vi "Simulation.CalcNextIteration.vi"(0 "Simulation in":refnum<class "Simulation.lvclass">, 1 "SimMode":T1, 5 "error in (no error)":errorcluster) -> (14 "Simulation out":refnum<class "Simulation.lvclass">, 19 "error out":errorcluster)   [LabVIEW 2016, in "Simulation.lvclass"]
uses:
  Simulation.lvclass
  SimModes.ctl
  Simulation.lvclass/Simulation.ctl
  Modell/Sondenmodell/Sondenmodell.lvclass/Sondenmodell.ctl
  Modell/Hausmodell/Hausmodell.lvclass/Hausmodell.ctl
  Modell/Umgebung/Umgebung.lvclass/Umgebung.ctl
  Modell/Hausmodell/Hausmodell.lvclass
  Modell/Sondenmodell/Sondenmodell.lvclass
  Modell/Umgebung/Umgebung.lvclass
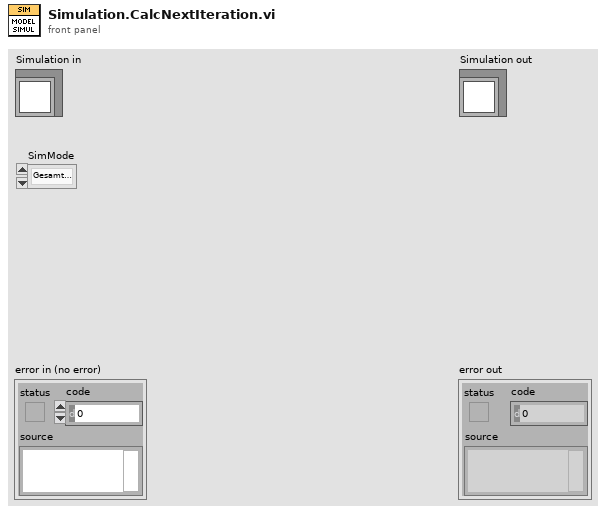
[diagram p1: front panel]
types:
  T1 = typedef "Simulation.lvclass/SimModes.ctl" = enum16{"Gesamtmodell", "HausOnly", "SondeOnly", "WPOnly"}
  T2 = typedef "Sondenmodell.lvclass/Sondenmodell.Zustandsgrössen.ctl" = cluster{"Erdtemperatur [°C]":dbl, "Rücklauftemperatur Solekreislauf [°C]":dbl}
  T3 = typedef "Hausmodell.lvclass/Hausmodell.Zustandsgrössen.ctl" = cluster{"Raumtemperatur [°C]":dbl, "Bodentemperatur [°C]":dbl, "Rücklauftemperatur Heizkreislauf [°C]":dbl}
  T4 = typedef "Umgebung.lvclass/Umgebung.Zustandsgrössen.ctl" = cluster{"Aussentemperatur [°C]":dbl, "Aussentemperatur [°C] Manuell":dbl, "Tag":dbl, "Stunde":dbl, "Minute":dbl, "Sekunden":dbl, "Strahlungsleistung [W/m2]":dbl, "Solare Gewinne [W/m2]":dbl, "Solare Gewinne [W/m2] Manuell":dbl, "Manuelle Eingabe On/Off":bool}
  T5 = typedef "Wärmepumpe.lvclass/Wärmepumpe.Zustandsgrössen.ctl" = cluster{"Vorlauftemperatur Heizkreislauf[°C]":dbl, "Vorlauftemperatur Solekreislauf[°C]":dbl, "Heizleistung [W]":dbl, "Kälteleistung [W]":dbl, "Verdichter 1":bool, "Verdichter 2":bool}
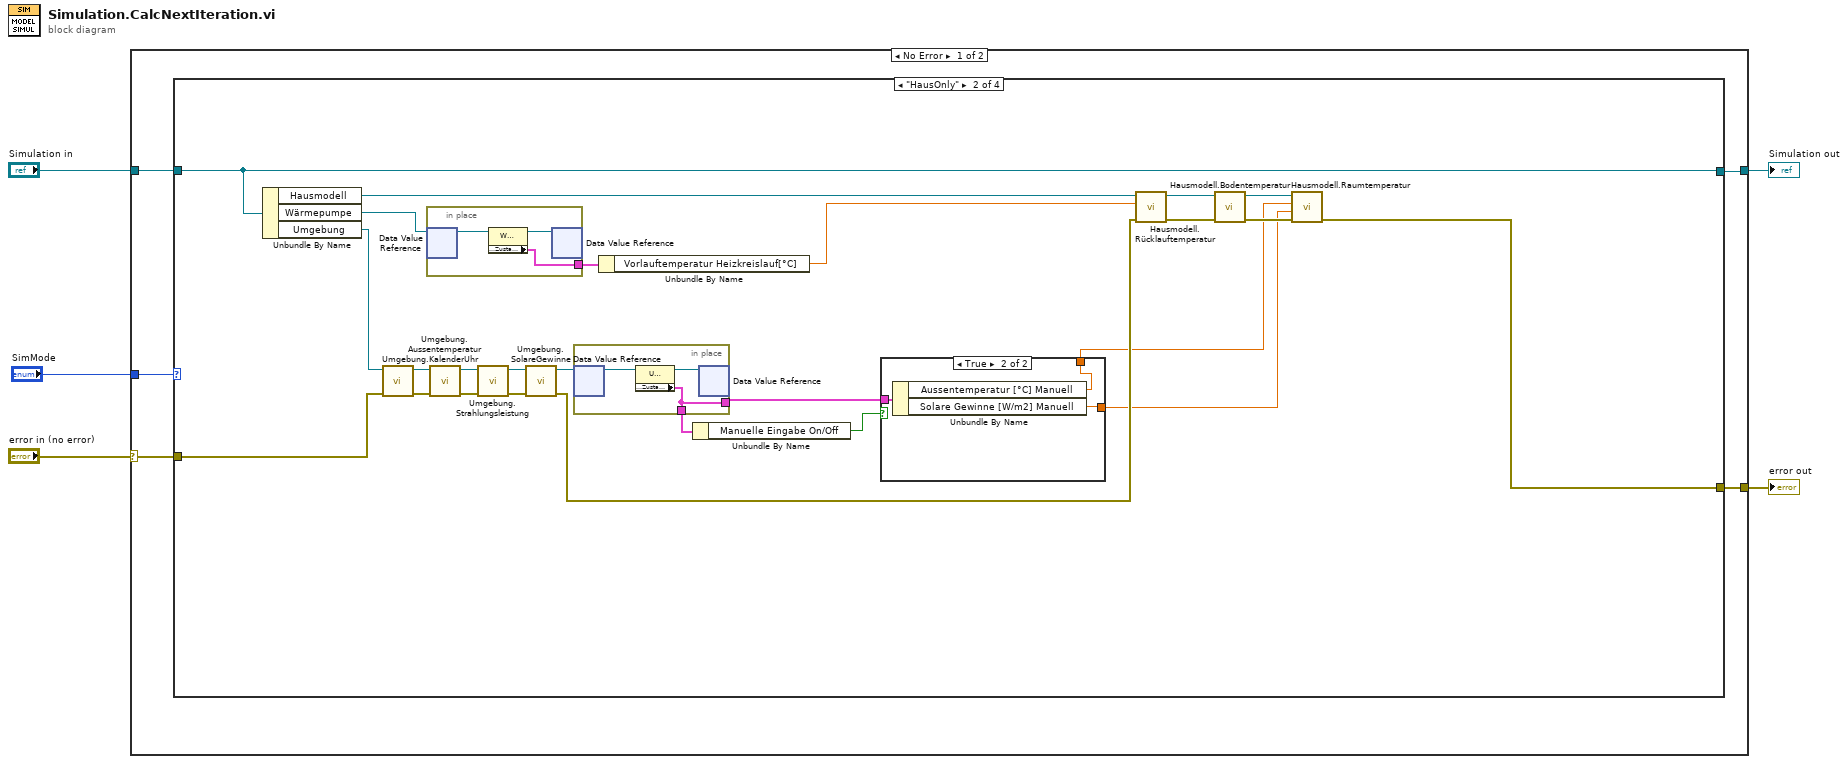
[diagram p0: block diagram]
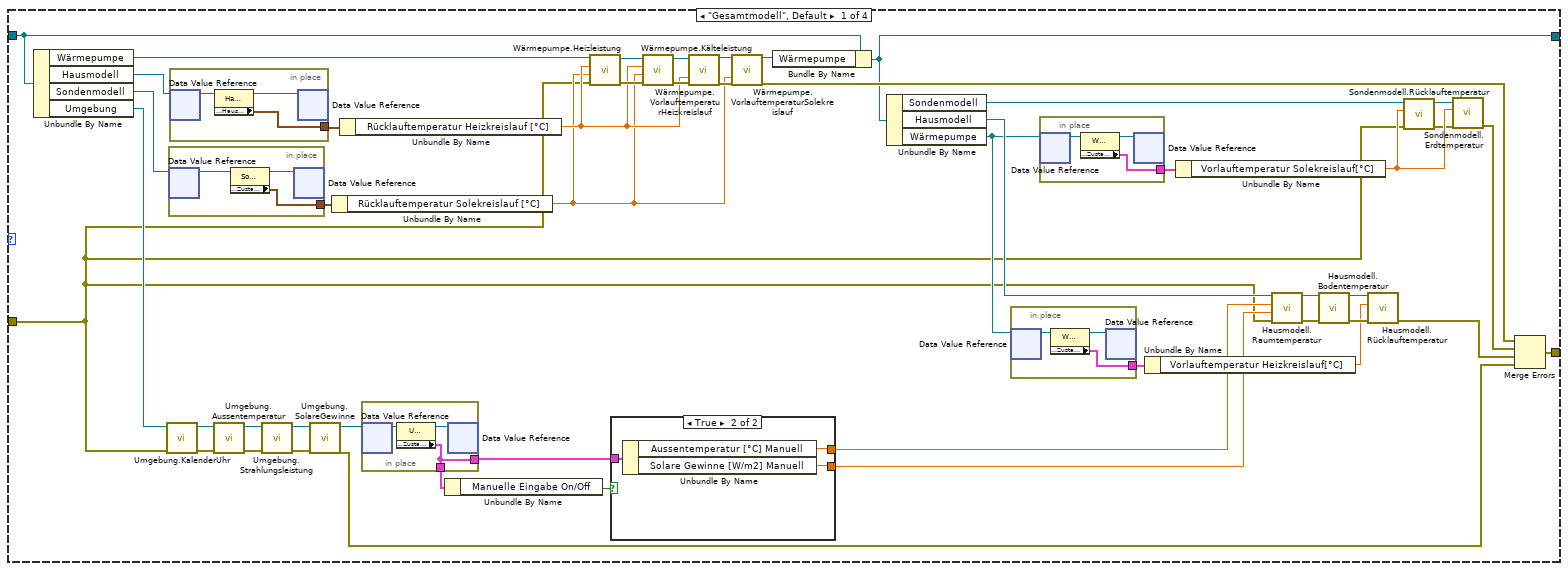
[diagram p2: hidden frame]
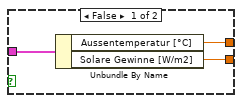
[diagram p3: hidden frame]
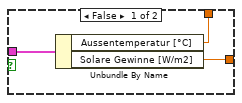
[diagram p4: hidden frame]
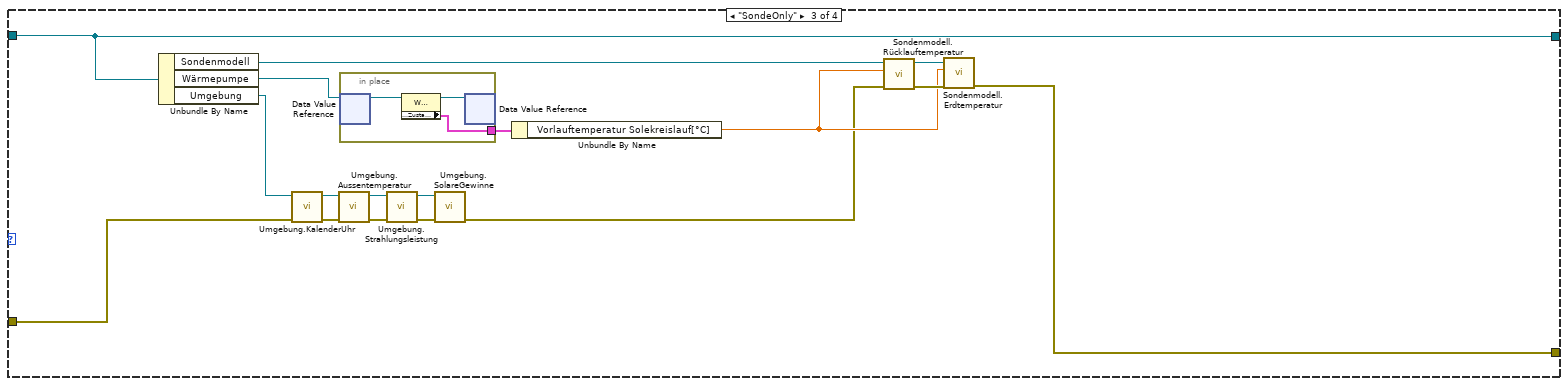
[diagram p5: hidden frame]
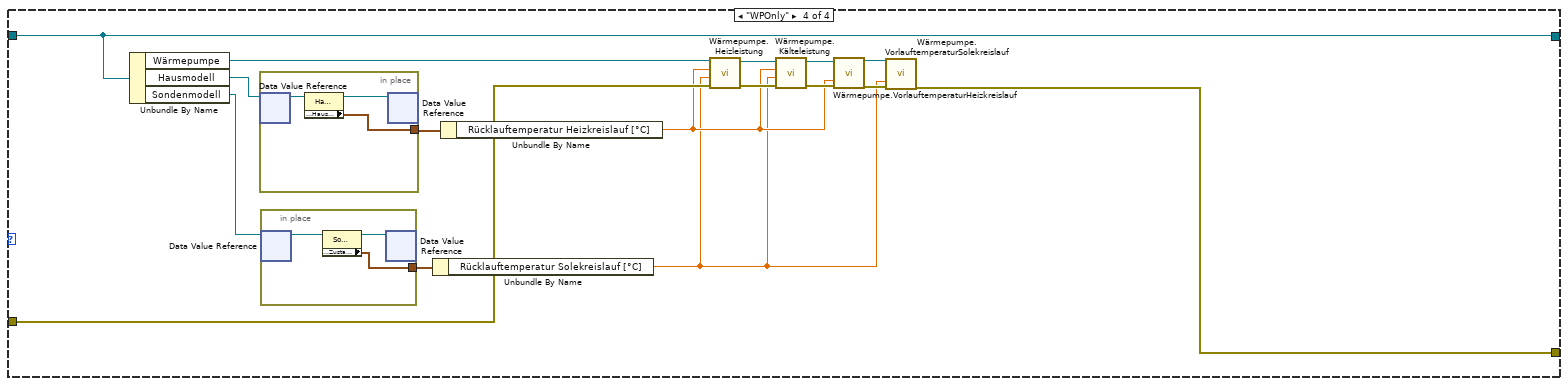
[diagram p6: hidden frame]
diagram:
  n1 = case shown="No Error" "error in (no error)" {
    selector: "error in (no error)" -> [w10 w160]
    tunnel: [w8 w160] -> w4
    tunnel: [w9 w159] -> w2
    tunnel: "Simulation in" -> [w7 w159]
    tunnel: "SimMode" -> [w6 _]
    frame No Error {
      n2 = case shown="\"HausOnly\"" w6 {
        tunnel: w10 -> [w13 w101 w118 w141]
        tunnel: [w23 w104 w131 w150] -> w9
        tunnel: [w34 w89 w127 w139] -> w8
        tunnel: w7 -> [w24 w104 w131 w150]
        frame "Gesamtmodell", Default {
          n3 = Unbundle By Name(w24) -> ("Wärmepumpe"=w50:refnum<data-value>, "Hausmodell"=w58:refnum<data-value>, "Sondenmodell"=w57:refnum<data-value>, "Umgebung"=w35:refnum<data-value>)
          n4 = call "Umgebung.KalenderUhr.vi"("Error in"=w13, "Umgebung in"=w35) -> ("Error out"=w42:errorcluster, "Umgebung out"=w45:refnum<data-value>)  [unwired: 8 in]
          n5 = in-place {
            in-place-border: [w74] -> w52
            n6 = in-place-dvr #1(w57) -> (w76:refnum<class "Sondenmodell.lvclass">)  [unwired: 1 out]
            n7 = property class="Sondenmodell.lvclass"(reference=w76) -> (reference out=w75:refnum<class "Sondenmodell.lvclass">, "Accessors:Sondenmodell.Zustandsgrössen"=w74:T2)  [unwired: 1 in, 1 out]
            n8 = in-place-dvr #1(w75) -> ()  [unwired: 2 out]
          }
          n9 = in-place {
            in-place-border: [w77] -> w51
            n10 = in-place-dvr #2(w58) -> (w79:refnum<class "Hausmodell.lvclass">)  [unwired: 1 out]
            n11 = property class="Hausmodell.lvclass"(reference=w79) -> (reference out=w78:refnum<class "Hausmodell.lvclass">, "Accessors:Zustandsgrössen.Hausmodell"=w77:T3)  [unwired: 1 in, 1 out]
            n12 = in-place-dvr #2(w78) -> ()  [unwired: 2 out]
          }
          n13 = call "Umgebung.Aussentemperatur.vi"("Error in"=w42, "Umgebung in"=w45) -> ("Error out"=w41:errorcluster, "Umgebung out"=w44:refnum<data-value>)  [unwired: 8 in]
          n14 = call "Umgebung.Strahlungsleistung.vi"("Error in"=w41, "Umgebung in"=w44) -> ("Error out"=w40:errorcluster, "Umgebung out"=w43:refnum<data-value>)  [unwired: 8 in]
          n15 = call "Umgebung.SolareGewinne.vi"("Error in"=w40, "Umgebung in"=w43) -> ("Error out"=w33:errorcluster, "Umgebung out"=w39:refnum<data-value>)  [unwired: 8 in]
          n16 = Unbundle By Name(w52) -> ("Rücklauftemperatur Solekreislauf [°C]"=w46:dbl)
          n17 = Unbundle By Name(w51) -> ("Rücklauftemperatur Heizkreislauf [°C]"=w47:dbl)
          n18 = in-place {
            in-place-border: [w71] -> w36
            in-place-border: [w71] -> w38
            n19 = in-place-dvr #3(w39) -> (w73:refnum<class "Umgebung.lvclass">)  [unwired: 1 out]
            n20 = property class="Umgebung.lvclass"(reference=w73) -> (reference out=w72:refnum<class "Umgebung.lvclass">, "Accessors:Umgebung.Zustandsgrössen"=w71:T4)  [unwired: 1 in, 1 out]
            n21 = in-place-dvr #3(w72) -> ()  [unwired: 2 out]
          }
          n22 = Unbundle By Name(w38) -> ("Manuelle Eingabe On/Off"=w37:bool)
          n23 = call "Wärmepumpe.Heizleistung.vi"("Error in"=w13, "Rücklauftemperatur Solekreislauf [°C]"=w46, "Rücklauftemperatur Heizkreislauf [°C]"=w47, "Wärmepumpe in"=w50) -> ("Error out"=w53:errorcluster, "Wärmepumpe out"=w54:refnum<data-value>)  [unwired: 6 in]
          n24 = case shown="True" w37 {
            tunnel: w36 -> [w67 w70]
            tunnel: [w66 w69] -> w21
            tunnel: [w65 w68] -> w20
            frame False {
              n25 = Unbundle By Name(w67) -> ("Aussentemperatur [°C]"=w65:dbl, "Solare Gewinne [W/m2]"=w66:dbl)
            }
            frame True {
              n26 = Unbundle By Name(w70) -> ("Aussentemperatur [°C] Manuell"=w68:dbl, "Solare Gewinne [W/m2] Manuell"=w69:dbl)
            }
          }
          n27 = call "Wärmepumpe.Kälteleistung.vi"("Error in"=w53, "Rücklauftemperatur Solekreislauf [°C]"=w46, "Rücklauftemperatur Heizkreislauf [°C]"=w47, "Wärmepumpe in"=w54) -> ("Error out"=w48:errorcluster, "Wärmepumpe out"=w49:refnum<data-value>)  [unwired: 6 in]
          n28 = call "Wärmepumpe.VorlauftemperaturHeizkreislauf.vi"("Wärmepumpe in"=w49, "Rücklauftemperatur  Heizkreislauf[°C]"=w47, "Error in"=w48) -> ("Wärmepumpe out"=w56:refnum<data-value>, "Error out"=w55:errorcluster)  [unwired: 15 in]
          n29 = call "Wärmepumpe.VorlauftemperaturSolekreislauf.vi"("Wärmepumpe in"=w56, "Rücklauftemperatur Solekreislauf[°C]"=w46, "Error in"=w55) -> ("Wärmepumpe out"=w25:refnum<data-value>, "Error out"=w32:errorcluster)  [unwired: 15 in]
          n30 = Bundle By Name(cluster=w24, "Wärmepumpe"=w25) -> (w23:refnum<class "Simulation.lvclass">)
          n31 = Unbundle By Name(w23) -> ("Sondenmodell"=w15:refnum<data-value>, "Hausmodell"=w22:refnum<data-value>, "Wärmepumpe"=w14:refnum<data-value>)
          n32 = in-place {
            in-place-border: [w62] -> w27
            n33 = in-place-dvr #4(w14) -> (w64:refnum<class "Wärmepumpe.lvclass">)  [unwired: 1 out]
            n34 = property class="Wärmepumpe.lvclass"(reference=w64) -> (reference out=w63:refnum<class "Wärmepumpe.lvclass">, "Accessors:Wärmepumpe.Zustandsgrössen"=w62:T5)  [unwired: 1 in, 1 out]
            n35 = in-place-dvr #4(w63) -> ()  [unwired: 2 out]
          }
          n36 = in-place {
            in-place-border: [w59] -> w16
            n37 = in-place-dvr #5(w14) -> (w61:refnum<class "Wärmepumpe.lvclass">)  [unwired: 1 out]
            n38 = property class="Wärmepumpe.lvclass"(reference=w61) -> (reference out=w60:refnum<class "Wärmepumpe.lvclass">, "Accessors:Wärmepumpe.Zustandsgrössen"=w59:T5)  [unwired: 1 in, 1 out]
            n39 = in-place-dvr #5(w60) -> ()  [unwired: 2 out]
          }
          n40 = Unbundle By Name(w27) -> ("Vorlauftemperatur Heizkreislauf[°C]"=w26:dbl)
          n41 = Unbundle By Name(w16) -> ("Vorlauftemperatur Solekreislauf[°C]"=w19:dbl)
          n42 = call "Hausmodell.Raumtemperatur.vi"("Error IN"=w13, "Solare Gewinne [W/m2]"=w21, "Aussentemperatur [°C]"=w20, "Hausmodell IN"=w22) -> ("Error OUT"=w31:errorcluster, "Hausmodell OUT"=w28:refnum<data-value>)  [unwired: 6 in]
          n43 = call "Hausmodell.Bodentemperatur.vi"("Error IN"=w31, "Hausmodell IN"=w28) -> ("Error OUT"=w30:errorcluster, "Hausmodell OUT"=w29:refnum<data-value>)  [unwired: 6 in]
          n44 = call "Hausmodell.Rücklauftemperatur.vi"("Error IN"=w30, "Vorlauftemperatur Heizkreislauf [°C]"=w26, "Hausmodell IN"=w29) -> ("Error OUT"=w11:errorcluster)  [unwired: 7 in, 1 out]
          n45 = call "Sondenmodell.Rücklauftemperatur.vi"("Error in"=w13, "Vorlauftemperatur Solekreislauf [°C]"=w19, "Sondenmodell in"=w15) -> ("Error out"=w18:errorcluster, "Sondenmodell out"=w17:refnum<data-value>)  [unwired: 7 in]
          n46 = call "Sondenmodell.Erdtemperatur.vi"("Error in"=w18, "Vorlauftemperatur Solekreislauf [°C]"=w19, "Sondenmodell in"=w17) -> ("Error out"=w12:errorcluster)  [unwired: 7 in, 1 out]
          n47 = Merge Errors(w32, w12, w11, w33) -> (w34:errorcluster)
        }
        frame "HausOnly" {
          n48 = Unbundle By Name(w104) -> ("Hausmodell"=w85:refnum<data-value>, "Wärmepumpe"=w103:refnum<data-value>, "Umgebung"=w100:refnum<data-value>)
          n49 = call "Umgebung.KalenderUhr.vi"("Error in"=w101, "Umgebung in"=w100) -> ("Error out"=w96:errorcluster, "Umgebung out"=w99:refnum<data-value>)  [unwired: 8 in]
          n50 = in-place {
            in-place-border: [w114] -> w102
            n51 = in-place-dvr #6(w103) -> (w116:refnum<class "Wärmepumpe.lvclass">)  [unwired: 1 out]
            n52 = property class="Wärmepumpe.lvclass"(reference=w116) -> (reference out=w115:refnum<class "Wärmepumpe.lvclass">, "Accessors:Wärmepumpe.Zustandsgrössen"=w114:T5)  [unwired: 1 in, 1 out]
            n53 = in-place-dvr #6(w115) -> ()  [unwired: 2 out]
          }
          n54 = call "Umgebung.Aussentemperatur.vi"("Error in"=w96, "Umgebung in"=w99) -> ("Error out"=w95:errorcluster, "Umgebung out"=w98:refnum<data-value>)  [unwired: 8 in]
          n55 = call "Umgebung.Strahlungsleistung.vi"("Error in"=w95, "Umgebung in"=w98) -> ("Error out"=w94:errorcluster, "Umgebung out"=w97:refnum<data-value>)  [unwired: 8 in]
          n56 = call "Umgebung.SolareGewinne.vi"("Error in"=w94, "Umgebung in"=w97) -> ("Error out"=w86:errorcluster, "Umgebung out"=w93:refnum<data-value>)  [unwired: 8 in]
          n57 = in-place {
            in-place-border: [w111] -> w90
            in-place-border: [w111] -> w92
            n58 = in-place-dvr #7(w93) -> (w113:refnum<class "Umgebung.lvclass">)  [unwired: 1 out]
            n59 = property class="Umgebung.lvclass"(reference=w113) -> (reference out=w112:refnum<class "Umgebung.lvclass">, "Accessors:Umgebung.Zustandsgrössen"=w111:T4)  [unwired: 1 in, 1 out]
            n60 = in-place-dvr #7(w112) -> ()  [unwired: 2 out]
          }
          n61 = Unbundle By Name(w102) -> ("Vorlauftemperatur Heizkreislauf[°C]"=w82:dbl)
          n62 = Unbundle By Name(w92) -> ("Manuelle Eingabe On/Off"=w91:bool)
          n63 = case shown="True" w91 {
            tunnel: w90 -> [w107 w110]
            tunnel: [w106 w109] -> w81
            tunnel: [w105 w108] -> w80
            frame False {
              n64 = Unbundle By Name(w107) -> ("Aussentemperatur [°C]"=w106:dbl, "Solare Gewinne [W/m2]"=w105:dbl)
            }
            frame True {
              n65 = Unbundle By Name(w110) -> ("Aussentemperatur [°C] Manuell"=w109:dbl, "Solare Gewinne [W/m2] Manuell"=w108:dbl)
            }
          }
          n66 = call "Hausmodell.Rücklauftemperatur.vi"("Error IN"=w86, "Vorlauftemperatur Heizkreislauf [°C]"=w82, "Hausmodell IN"=w85) -> ("Error OUT"=w87:errorcluster, "Hausmodell OUT"=w84:refnum<data-value>)  [unwired: 7 in]
          n67 = call "Hausmodell.Bodentemperatur.vi"("Error IN"=w87, "Hausmodell IN"=w84) -> ("Error OUT"=w88:errorcluster, "Hausmodell OUT"=w83:refnum<data-value>)  [unwired: 6 in]
          n68 = call "Hausmodell.Raumtemperatur.vi"("Error IN"=w88, "Solare Gewinne [W/m2]"=w80, "Aussentemperatur [°C]"=w81, "Hausmodell IN"=w83) -> ("Error OUT"=w89:errorcluster)  [unwired: 6 in, 1 out]
        }
        frame "SondeOnly" {
          n69 = Unbundle By Name(w131) -> ("Sondenmodell"=w130:refnum<data-value>, "Wärmepumpe"=w133:refnum<data-value>, "Umgebung"=w119:refnum<data-value>)
          n70 = call "Umgebung.KalenderUhr.vi"("Error in"=w118, "Umgebung in"=w119) -> ("Error out"=w122:errorcluster, "Umgebung out"=w125:refnum<data-value>)  [unwired: 8 in]
          n71 = call "Umgebung.Aussentemperatur.vi"("Error in"=w122, "Umgebung in"=w125) -> ("Error out"=w121:errorcluster, "Umgebung out"=w124:refnum<data-value>)  [unwired: 8 in]
          n72 = in-place {
            in-place-border: [w134] -> w132
            n73 = in-place-dvr #8(w133) -> (w136:refnum<class "Wärmepumpe.lvclass">)  [unwired: 1 out]
            n74 = property class="Wärmepumpe.lvclass"(reference=w136) -> (reference out=w135:refnum<class "Wärmepumpe.lvclass">, "Accessors:Wärmepumpe.Zustandsgrössen"=w134:T5)  [unwired: 1 in, 1 out]
            n75 = in-place-dvr #8(w135) -> ()  [unwired: 2 out]
          }
          n76 = call "Umgebung.Strahlungsleistung.vi"("Error in"=w121, "Umgebung in"=w124) -> ("Error out"=w120:errorcluster, "Umgebung out"=w123:refnum<data-value>)  [unwired: 8 in]
          n77 = call "Umgebung.SolareGewinne.vi"("Error in"=w120, "Umgebung in"=w123) -> ("Error out"=w117:errorcluster)  [unwired: 8 in, 1 out]
          n78 = Unbundle By Name(w132) -> ("Vorlauftemperatur Solekreislauf[°C]"=w126:dbl)
          n79 = call "Sondenmodell.Rücklauftemperatur.vi"("Error in"=w117, "Vorlauftemperatur Solekreislauf [°C]"=w126, "Sondenmodell in"=w130) -> ("Error out"=w128:errorcluster, "Sondenmodell out"=w129:refnum<data-value>)  [unwired: 7 in]
          n80 = call "Sondenmodell.Erdtemperatur.vi"("Error in"=w128, "Vorlauftemperatur Solekreislauf [°C]"=w126, "Sondenmodell in"=w129) -> ("Error out"=w127:errorcluster)  [unwired: 7 in, 1 out]
        }
        frame "WPOnly" {
          n81 = Unbundle By Name(w150) -> ("Wärmepumpe"=w143:refnum<data-value>, "Hausmodell"=w152:refnum<data-value>, "Sondenmodell"=w151:refnum<data-value>)
          n82 = in-place {
            in-place-border: [w156] -> w144
            n83 = in-place-dvr #9(w152) -> (w158:refnum<class "Hausmodell.lvclass">)  [unwired: 1 out]
            n84 = property class="Hausmodell.lvclass"(reference=w158) -> (reference out=w157:refnum<class "Hausmodell.lvclass">, "Accessors:Zustandsgrössen.Hausmodell"=w156:T3)  [unwired: 1 in, 1 out]
            n85 = in-place-dvr #9(w157) -> ()  [unwired: 2 out]
          }
          n86 = in-place {
            in-place-border: [w153] -> w145
            n87 = in-place-dvr #10(w151) -> (w155:refnum<class "Sondenmodell.lvclass">)  [unwired: 1 out]
            n88 = property class="Sondenmodell.lvclass"(reference=w155) -> (reference out=w154:refnum<class "Sondenmodell.lvclass">, "Accessors:Sondenmodell.Zustandsgrössen"=w153:T2)  [unwired: 1 in, 1 out]
            n89 = in-place-dvr #10(w154) -> ()  [unwired: 2 out]
          }
          n90 = Unbundle By Name(w145) -> ("Rücklauftemperatur Solekreislauf [°C]"=w137:dbl)
          n91 = Unbundle By Name(w144) -> ("Rücklauftemperatur Heizkreislauf [°C]"=w138:dbl)
          n92 = call "Wärmepumpe.Heizleistung.vi"("Error in"=w141, "Rücklauftemperatur Solekreislauf [°C]"=w137, "Rücklauftemperatur Heizkreislauf [°C]"=w138, "Wärmepumpe in"=w143) -> ("Error out"=w146:errorcluster, "Wärmepumpe out"=w147:refnum<data-value>)  [unwired: 6 in]
          n93 = call "Wärmepumpe.Kälteleistung.vi"("Error in"=w146, "Rücklauftemperatur Solekreislauf [°C]"=w137, "Rücklauftemperatur Heizkreislauf [°C]"=w138, "Wärmepumpe in"=w147) -> ("Error out"=w140:errorcluster, "Wärmepumpe out"=w142:refnum<data-value>)  [unwired: 6 in]
          n94 = call "Wärmepumpe.VorlauftemperaturHeizkreislauf.vi"("Wärmepumpe in"=w142, "Rücklauftemperatur  Heizkreislauf[°C]"=w138, "Error in"=w140) -> ("Wärmepumpe out"=w149:refnum<data-value>, "Error out"=w148:errorcluster)  [unwired: 15 in]
          n95 = call "Wärmepumpe.VorlauftemperaturSolekreislauf.vi"("Wärmepumpe in"=w149, "Rücklauftemperatur Solekreislauf[°C]"=w137, "Error in"=w148) -> ("Error out"=w139:errorcluster)  [unwired: 15 in, 1 out]
        }
      }
    }
    frame Error {
    }
  }
  "error out" <- w4
  "Simulation out" <- w2
